vi "Read Trace Data.vi"(8 "error in (no error)":errorcluster, 10 "Count Value (1)":i32=1, 11 "VISA resource name":refnum<visa-resource-name>) -> (0 "error out":errorcluster, 2 "Measurements":T1(array[cluster]) {"Measurement" format="%.6e"}, 3 "VISA resource name out":refnum<visa-resource-name>)   [LabVIEW 2019, in "Keithley 6517.lvlib"]
doc: "Returns the specified measurement data in the trace buffer."
uses:
  Keithley 6517.lvlib
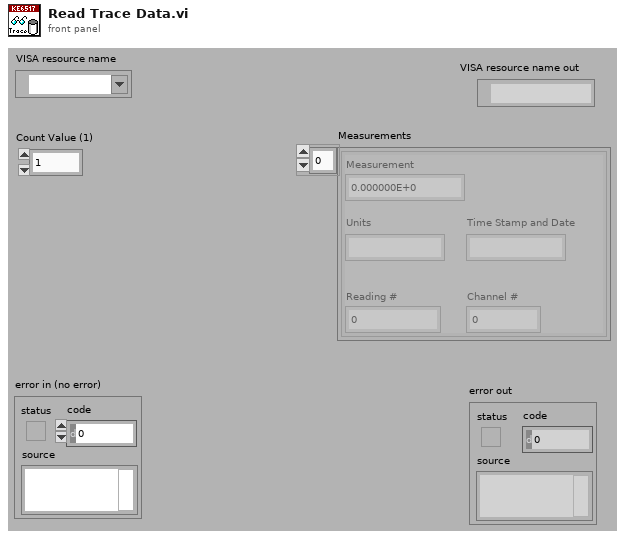
[diagram p1: front panel]
types:
  T1 = cluster{"Measurement":dbl, "Units":string, "Time Stamp and Date":string, "Reading #":dbl, "Channel #":dbl}[]
  T2 = typedef "Keithley 6517.lvlib/Extended User Data.ctl" = cluster{"Instrument Model":i32}
  T3 = cluster{"Measurement":dbl, "Units":string, "Time Stamp and Date":string, "Reading #":dbl, "Channel #":dbl}
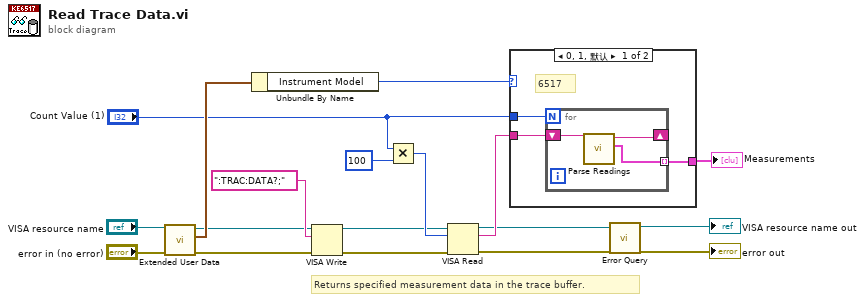
[diagram p0: block diagram]
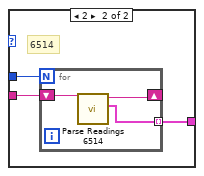
[diagram p2: hidden frame]
diagram:
  # "Returns specified measurement data in the trace buffer."
  n1 = call "Extended User Data.vi"("error in (no error)"="error in (no error)", "VISA resource name"="VISA resource name") -> ("error out"=w9:errorcluster, "User Data Out"=w11:T2, "VISA resource name out"=w10:refnum<visa-resource-name>)  [unwired: 7 in]
  n2 = Unbundle By Name(w11) -> ("Instrument Model"=w8:i32)
  n3 = VISA Write(VISA resource name=w10, write buffer=":TRAC:DATA?;", error in (no error)=w9) -> (VISA resource name out=w7:refnum<visa-resource-name>, error out=w6:errorcluster)  [unwired: 1 out]
  n4 = Multiply(x="Count Value (1)", y=u32 100 ("byte count")) -> (x*y=w14:u32)
  n5 = VISA Read(VISA resource name=w7, byte count=w14, error in (no error)=w6) -> (VISA resource name out=w3:refnum<visa-resource-name>, read buffer=w4:string, error out=w2:errorcluster)  [unwired: 1 out]
  n6 = case shown="0, 1, 默认" w8 {
    tunnel: "Count Value (1)" -> [w21 w27]
    tunnel: w4 -> [w20 w26]
    tunnel: [w19 w25] -> w1
    frame 0, 1, Default {
      # "6517"
      n7 = for {
        N: w21 -> [_]
        shift-right: [w22] -> _
        shift-left: w20 -> [w24]
        tunnel: [w23] -> w19 mode=indexing
        n8 = call "Parse Readings.vi"("Readings"=w24) -> ("Measurement"=w23:T3, "Remain Readings"=w22:string)  [unwired: 9 in]
      }
    }
    frame 2 {
      # "6514"
      n9 = for {
        N: w27 -> [_]
        shift-right: [w28] -> _
        shift-left: w26 -> [w30]
        tunnel: [w29] -> w25 mode=indexing
        n10 = call "Parse Readings 6514.vi"("Readings"=w30) -> ("Measurement"=w29:T3, "Remain Readings"=w28:string)  [unwired: 9 in]
      }
    }
  }
  "Measurements" <- w1
  n11 = call "Error Query.vi"("error in (no error)"=w2, "VISA resource name"=w3) -> ("error out"=→"error out":errorcluster, "VISA resource name out"=→"VISA resource name out":refnum<visa-resource-name>)  [unwired: 6 in, 2 out]
